vi "TAT_PLC_Data_read_BOLLEAN.vi"(7 "Enum":enum16{"Read", "Write"}(ring), 8 "error in (no error)":errorcluster, 10 "Array":bool[](array[boolean])) -> (0 "error out":errorcluster, 2 "Array 2":bool[](array[boolean]))   [LabVIEW 2017]
panel:
  # "STATION 1\nand\nSTATION 2"
  # "SR.NO\tFROM PLC TO SOFTWARE\tDESCRIPTION\tTO SOFTWARE\n1\tM110\tPLC HEALTHY\t8302\n2\tM111\tAUTO CYCLE START\t8303\n3\tM112\tSPARE\t8304\n4\tM113\tAUTO CYCLE COMPLETE\t8305\n5\tM114\tSTATION 1 SCANNING START\t8306\n6\tM115\tSTATION 1 DATA SAVE\t8307\n7\tM116\tSTATION 2 SCANNING START\t8308\n8\tM117\tSTATION 2 DATA SAVE\t8309"
  # "CONTROL PROCESS TO  LABVIEW from PLC"
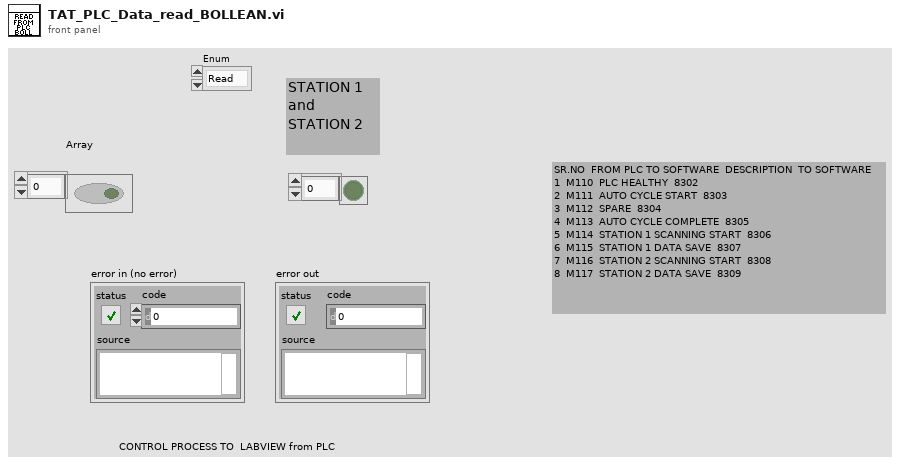
[diagram p1: front panel]
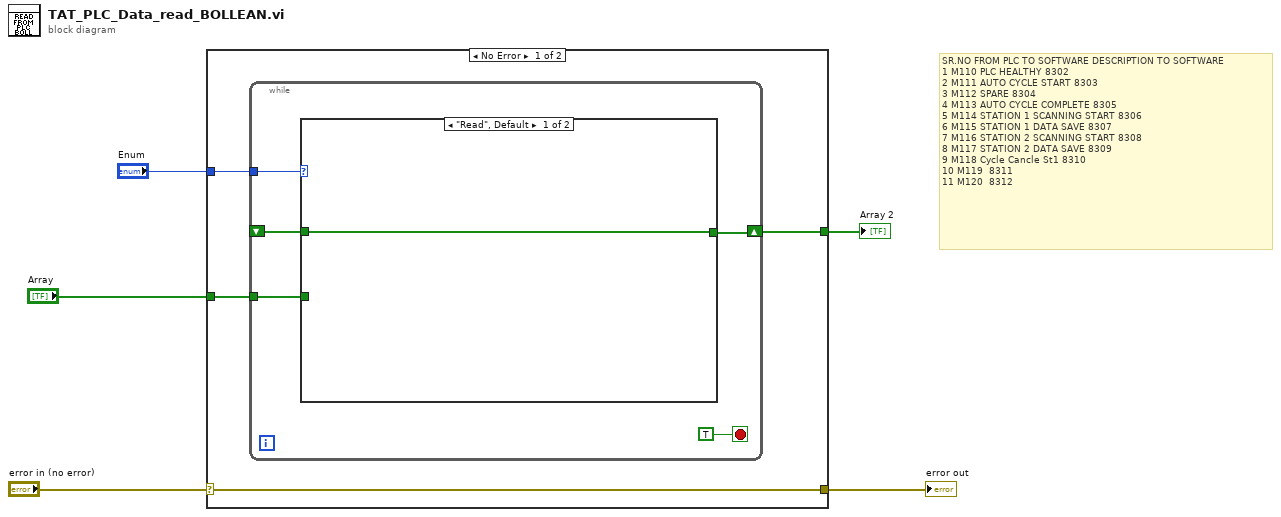
[diagram p0: block diagram]
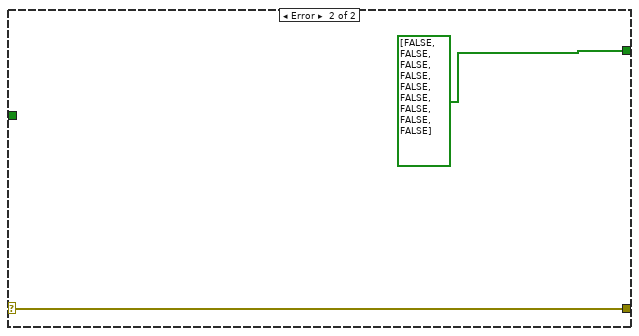
[diagram p3: hidden frame]
diagram:
  # "SR.NO\tFROM PLC TO SOFTWARE\tDESCRIPTION\tTO SOFTWARE\n1\tM110\tPLC HEALTHY\t8302\n2\tM111\tAUTO CYCLE START\t8303\n3\tM112\tSPARE\t8304\n4\tM113\tAUTO CYCLE COMPLETE\t8305\n5\tM114\tSTATION 1 SCANNING START\t8306\n6\tM115\tSTATION 1 DATA SAVE\t8307\n7\tM116\tSTATION 2 SCANNING START\t8308\n8\tM117\tSTATION 2 DATA SAVE\t8309\n9\tM118\tCycle Cancle St1\t8310\n10\tM119\t\t8311\n11\tM120\t\t8312"
  n1 = case shown="No Error" "error in (no error)" {
    selector: "error in (no error)" -> [w6 w18]
    tunnel: [w6 w18] -> w5
    tunnel: "Enum" -> [w9 _]
    tunnel: "Array" -> [w8 _]
    tunnel: [w7 bool[] [FALSE, FALSE, FALSE, FALSE, FALSE, FALSE, FALSE, FALSE, FALSE]] -> w1
    frame No Error {
      n2 = while {
        tunnel: w9 -> [w13]
        shift-right: [w10] -> w7
        shift-left: _ -> [w11]
        tunnel: w8 -> [w12]
        stop <- TRUE stop-if-true
        n3 = case shown="\"Read\", Default" w13 {
          tunnel: w12 -> [_ w16]
          tunnel: [w15 w16] -> w10
          tunnel: w11 -> [w15 _]
          frame "Read", Default {
          }
          frame "Write" {
          }
        }
      }
    }
    frame Error {
    }
  }
  "error out" <- w5
  "Array 2" <- w1
